vi "ROS_Topic_Read.vi"(2 "Timeout (ms)":i32=5000, 3 "ROS in":T1={"topic port"=0, "Node"="", "topic"="", "type"="", "node port"=0, "error "={"status"=FALSE, "code"=0, "source"=""}, "Direction"=enum."Node", "APIs"=[], "Update (ms)"=1, "write queue"=1}) -> (0 "Reply":string, 1 "ROS out":T1={"topic port"=0, "Node"="", "topic"="", "type"="", "node port"=0, "error "={"status"=FALSE, "code"=0, "source"=""}, "Direction"=enum."Node", "APIs"=[], "Update (ms)"=1, "write queue"=1})   [LabVIEW 2010]
doc: "Waits for a non-empty message on the ROS topic or service until Timeout."
uses:
  <userlib>/ROSforLV/ROS/Code/SubVIs/_ROSControl.ctl
  <userlib>/ROSforLV/ROS/Code/SubVIs/_ROSDirection.ctl
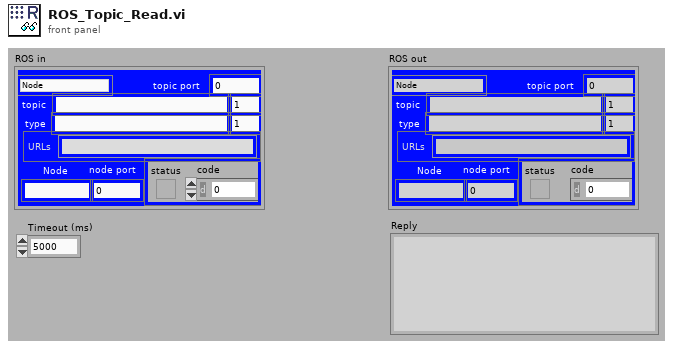
[diagram p1: front panel]
types:
  T1 = typedef "_ROSControl.ctl" = cluster{"topic port":u16, "Node":string, "topic":string, "type":string, "node port":u32, "error ":errorcluster, "Direction":T2, "APIs":string[], "Update (ms)":u16, "write queue":u16}
  T2 = typedef "_ROSDirection.ctl" = enum16{"Node", "Publisher", "Subscriber", "Service Client"}
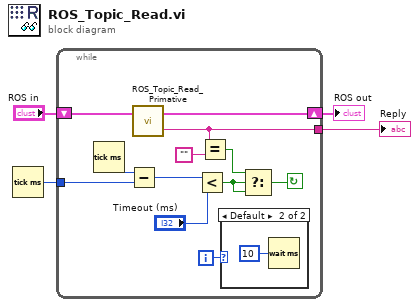
[diagram p0: block diagram]
diagram:
  n1 = Tick Count (ms)() -> (millisecond timer value=w1:u32)
  n2 = while {
    shift-right: [w15] -> w3
    shift-left: "ROS in" -> [w14]
    tunnel: [w13] -> w2
    tunnel: w1 -> [w11]
    i -> [w5]
    stop <- w7 continue-if-true
    n3 = Tick Count (ms)() -> (millisecond timer value=w12:u32)
    n4 = Subtract(x=w12, y=w11) -> (x-y=w10:u32)
    n5 = call <userlib>:"ROS_Topic_Read_Primative.vi"("ROS in"=w14) -> ("Reply"=w13:string, "ROS out"=w15:T1)  [unwired: 1 in]
    n6 = Less?(x=w10, y="Timeout (ms)") -> (x < y?=w9:bool)
    n7 = Equal?(x=w13, y="") -> (x = y?=w8:bool)
    n8 = case shown="Default" w5 {
      frame 0 {
      }
      frame Default {
        n9 = Wait (ms)(milliseconds to wait=u32 10) -> ()  [unwired: 1 out]
      }
    }
    n10 = Select(t=w8, s=w9, f=w9) -> (s? t:f=w7:bool)
  }
  "ROS out" <- w3
  "Reply" <- w2
